vi "Check_Modbus_Packet_Header.vi"(8 "error in (no error)":errorcluster, 11 "VISA resource name":refnum<visa-resource-name>) -> (0 "error out":errorcluster, 1 "header_array":u8[](array[numeric]), 2 "Length":u8, 3 "VISA Refnum out":refnum<visa-resource-name>)   [LabVIEW 2026]
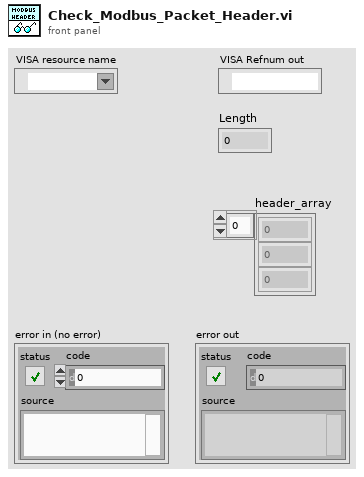
[diagram p1: front panel]
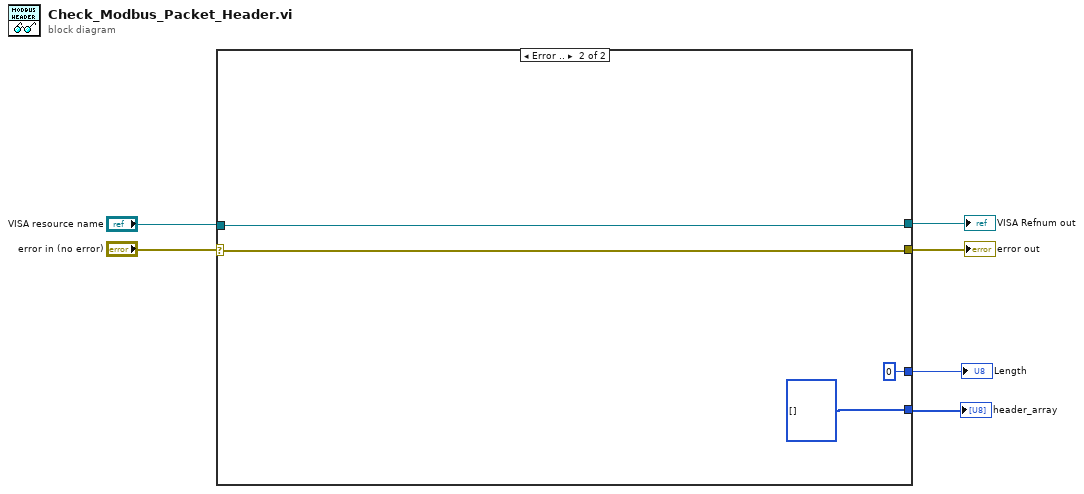
[diagram p0: block diagram]
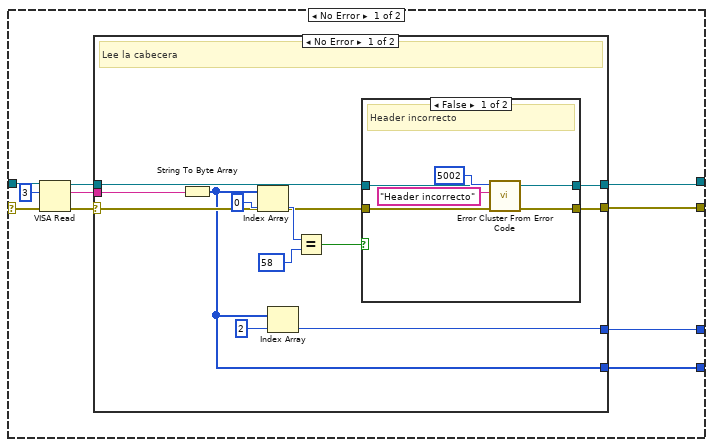
[diagram p2: hidden frame]
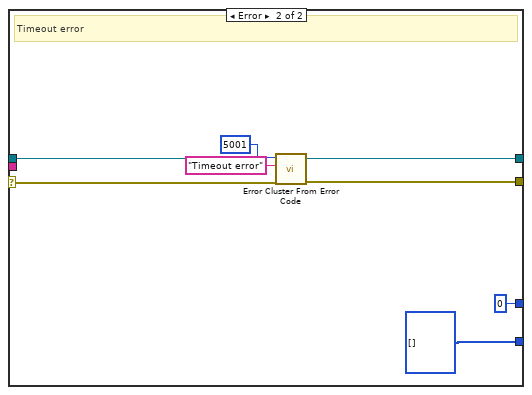
[diagram p4: hidden frame]
diagram:
  n1 = case shown="Error .." "error in (no error)" {
    selector: "error in (no error)" -> [w15 w45]
    tunnel: "VISA resource name" -> [w16 w46]
    tunnel: [w12 w45] -> w4
    tunnel: [w10 w46] -> w3
    tunnel: [w8 u8 0] -> w2
    tunnel: [w7 u8[] [] ("unsigned byte array")] -> w1
    frame No Error {
      n2 = VISA Read(VISA resource name=w16, byte count=u32 3, error in (no error)=w15) -> (VISA resource name out=w11:refnum<visa-resource-name>, read buffer=w9:string, error out=w13:errorcluster)  [unwired: 1 out]
      n3 = case shown="No Error" w13 {
        selector: w13 -> [w21 w42]
        tunnel: [w20 w41] -> w12
        tunnel: w11 -> [w23 w38]
        tunnel: [w22 w38] -> w10
        tunnel: w9 -> [w28 _]
        tunnel: [w18 u8 0] -> w8
        tunnel: [w17 u8[] [] ("unsigned byte array")] -> w7
        frame No Error {
          # "Lee la cabecera"
          n4 = String To Byte Array(string=w28) -> (unsigned byte array=w17:u8[])
          n5 = Index Array(array=w17, index=0) -> (element=w26:u8)
          n6 = Index Array(array=w17, index=2) -> (element=w18:u8)
          n7 = Equal?(x=w26, y=u8 58) -> (x = y?=w24:bool)
          n8 = case shown="False" w24 {
            tunnel: w23 -> [w29 w35]
            tunnel: [w29 w35] -> w22
            tunnel: w21 -> [w31 w34]
            tunnel: [w30 w34] -> w20
            frame False {
              # "Header incorrecto"
              n9 = call <vilib>:"Error Cluster From Error Code.vi"("error in (no error)"=w31, "error message (\"\")"="Header incorrecto" ("error message (\"\")"), "error code (0)"=5002) -> ("error out"=w30:errorcluster)  [unwired: 6 in]
            }
            frame True {
              # "Header correcto"
            }
          }
        }
        frame Error {
          # "Timeout error"
          n10 = call <vilib>:"Error Cluster From Error Code.vi"("error in (no error)"=w42, "error message (\"\")"="Timeout error" ("error message (\"\")"), "error code (0)"=5001) -> ("error out"=w41:errorcluster)  [unwired: 6 in]
        }
      }
    }
    frame Error {
    }
  }
  "VISA Refnum out" <- w3
  "error out" <- w4
  "Length" <- w2
  "header_array" <- w1
